vi "Set Status_IO.vi"(8 "error in (no error)":errorcluster, 10 "Status":T1={"Device Data"=variant(cluster{"DeviceName":string, "COM":refnum<visa-resource-name>, "Status String":string, "Input String":string, "DI Value ":i32}[] []), "Ordered ICP1-DO Channels"=[], "Ordered ICP2-DI Channels"=[], "Ordered ICP2-DO Channels"=[], "Ordered ICP1-AI Channels"=[], "Ordered ICP1-AO Channels"=[], "Ordered ICP2-AO Channels"=[]}, 11 "IO in":refnum<class "IO.lvclass">) -> (0 "error out":errorcluster, 3 "IO out":refnum<class "IO.lvclass">)   [LabVIEW 2022 SP3, in "IO.lvclass"]
uses:
  IO.lvclass
  Typedefs/Status Cluster.ctl
  Typedefs/ICP1-D0 Channel Names.ctl
  Typedefs/ICP2-DI Channel Names.ctl
  Typedefs/ICP2-DO Channel Names.ctl
  Typedefs/ICP1-AI Channel Names.ctl
  Typedefs/ICP1-AO Channel Names.ctl
  Typedefs/ICP2-AO Channel Names.ctl
  IO.lvclass/IO.ctl
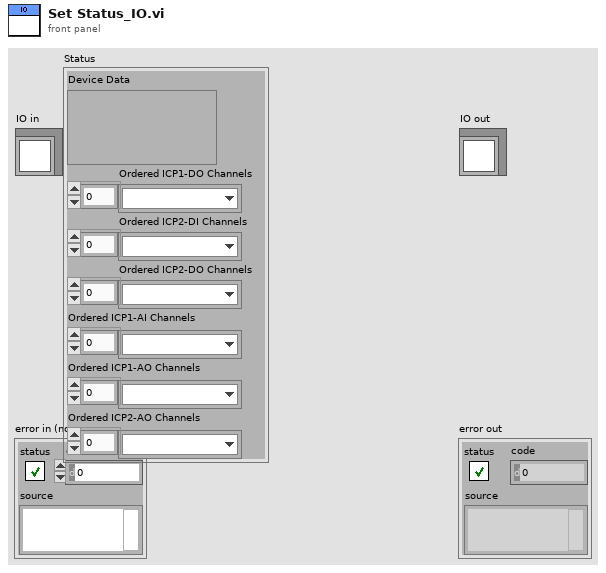
[diagram p1: front panel]
types:
  T1 = typedef "IO.lvclass/Status Cluster.ctl" = cluster{"Device Data":variant, "Ordered ICP1-DO Channels":T2[], "Ordered ICP2-DI Channels":T3[], "Ordered ICP2-DO Channels":T4[], "Ordered ICP1-AI Channels":T5[], "Ordered ICP1-AO Channels":T6[], "Ordered ICP2-AO Channels":T7[]}
  T2 = typedef "IO.lvclass/ICP1-D0 Channel Names.ctl" = enum16{"None", "Meniscus Pressure Reg PWR - R1", "Meniscus Pressure Reg PWR - R2", "Meniscus Pressure Reg PWR - R3", "Meniscus Pressure Reg PWR - R4", "Meniscus Pressure Reg PWR - R5", "Meniscus Pressure Reg PWR - R6", "Clear Stage Alarm", "Servo ON", "Purge Valve Open - R1", "Purge Valve Open - R2", "Purge Valve Open - R3", "Purge Valve Open - R4", "Purge Valve Open - R5", "Purge Valve Open - R6"}
  T3 = typedef "IO.lvclass/ICP2-DI Channel Names.ctl" = enum16{"None", "SW - Ink Valve - R1", "SW - Ink Valve - R2", "SW - Ink Valve - R3", "SW - Ink Valve - R4", "SW - Ink Valve - R5", "SW - Ink Valve - R6", "SW - COVER INPUT SIDE", "SW - COVER OUTPUT SIDE", "SW - Purge - R1", "SW - Purge - R2", "SW - Purge - R3", "SW - Purge - R4", "SW - Purge - R5", "SW - Purge - R6"}
  T4 = typedef "IO.lvclass/ICP2-DO Channel Names.ctl" = enum16{"None", "Meniscus Valve Open - R1", "Meniscus Valve Open - R2", "Meniscus Valve Open - R3", "Meniscus Valve Open - R4", "Meniscus Valve Open - R5", "Meniscus Valve Open - R6", "Ink Flow Valve Open - R1", "Ink Flow Valve Open - R2", "Ink Flow Valve Open - R3", "Ink Flow Valve Open - R4", "Ink Flow Valve Open - R5", "Ink Flow Valve Open - R6", "SW_LED - Ink Valve - R1", "SW_LED - Ink Valve - R2", "SW_LED - Ink Valve - R3", "Recirc Pump On - R1", "Recirc Pump On - R2", "Recirc Pump On - R3", "Recirc Pump On - R4", "Recirc Pump On - R5", "Recirc Pump On - R6", "SW_LED - Ink Valve - R4", "SW_LED - Ink Valve - R5", "SW_LED - Ink Valve - R6"}
  T5 = typedef "IO.lvclass/ICP1-AI Channel Names.ctl" = enum16{"None", "Meniscus Pressure Read - R1", "Meniscus Pressure Read - R2", "Meniscus Pressure Read - R3", "Meniscus Pressure Read - R4", "Meniscus Pressure Read - R5", "Meniscus Pressure Read - R6", "Meniscus Pressure Set - R1", "Meniscus Pressure Set - R2", "Meniscus Pressure Set - R3", "Meniscus Pressure Set - R4", "Meniscus Pressure Set - R5", "Meniscus Pressure Set - R6"}
  T6 = typedef "IO.lvclass/ICP1-AO Channel Names.ctl" = enum16{"None", "Meniscus Pressure Set - R1", "Meniscus Pressure Set - R2", "Meniscus Pressure Set - R3", "Meniscus Pressure Set - R4", "Meniscus Pressure Set - R5", "Meniscus Pressure Set - R6", "Meniscus Vac Pump Speed"}
  T7 = typedef "IO.lvclass/ICP2-AO Channel Names.ctl" = enum16{"None", "Recirc Pump Flow Set - R1", "Recirc Pump Flow Set - R2", "Recirc Pump Flow Set - R3", "Recirc Pump Flow Set - R4", "Recirc Pump Flow Set - R5", "Recirc Pump Flow Set - R6"}
  T8 = typedef "IO.lvclass/Private Data.ctl" = cluster{"UserEvents":T9, "All Dependencies":cluster{"Class References":refnum<class>[], "Class Names":string[]}, "Status":T1}
  T9 = typedef "IO.lvclass/UserEvents.ctl" = cluster{"API Incoming Event":refnum<user-event>, "API Executed Event":refnum<user-event>, "API Return Event":refnum<user-event>, "Status Changed Event":refnum<user-event>}
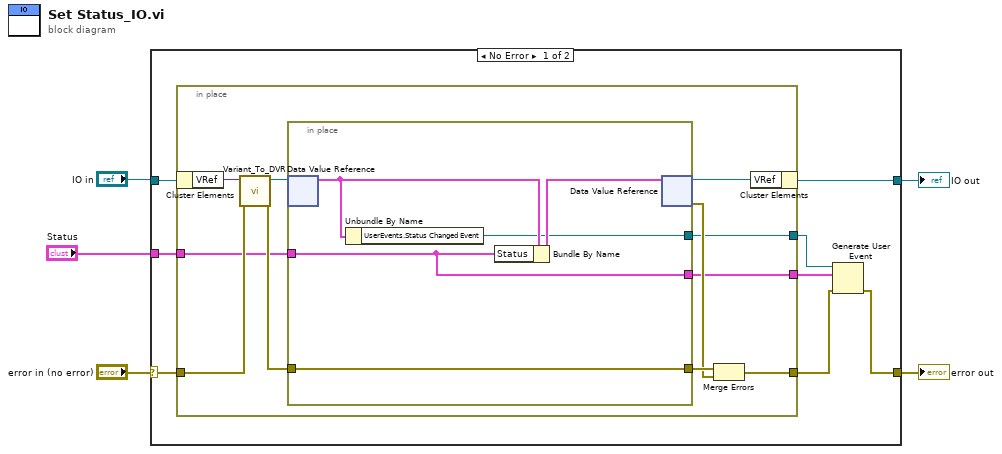
[diagram p0: block diagram]
diagram:
  n1 = case shown="No Error" "error in (no error)" {
    selector: "error in (no error)" -> [w11 w31]
    tunnel: [w6 w31] -> w3
    tunnel: [w13 w30] -> w2
    tunnel: "IO in" -> [w12 w30]
    tunnel: "Status" -> [w10 _]
    frame No Error {
      n2 = in-place {
        in-place-border: w11 -> [w22]
        in-place-border: [w18] -> w7
        in-place-border: w10 -> [w16]
        in-place-border: [w15] -> w9
        in-place-border: [w14] -> w8
        n3 = in-place-cluster #1(w12) -> ("VRef"=w24:variant)
        n4 = call "Variant_To_DVR.vi"("error in (no error)"=w22, "Variant"=w24) -> ("error out"=w21:errorcluster, "DVR"=w23:refnum<data-value>)  [unwired: 8 in]
        n5 = in-place {
          in-place-border: w21 -> [w29]
          in-place-border: [w29] -> w20
          in-place-border: w16 -> [w25]
          in-place-border: [w26] -> w15
          in-place-border: [w25] -> w14
          n6 = in-place-dvr #2(w23) -> (w27:T8)  [unwired: 1 out]
          n7 = Unbundle By Name(w27) -> ("UserEvents.Status Changed Event"=w26:refnum<user-event>)
          n8 = Bundle By Name(cluster=w27, "Status"=w25) -> (w28:T8)
          n9 = in-place-dvr #2(w28) -> (w17:refnum<data-value>, w19:errorcluster)
        }
        n10 = Merge Errors(w20, w19) -> (w18:errorcluster)
        n11 = in-place-cluster #1("VRef"=w17) -> (w13:refnum<class "IO.lvclass">)
      }
      n12 = Generate User Event(user event=w9, event data cluster=w8, error in=w7) -> (error out=w6:errorcluster)  [unwired: 1 in, 1 out]
    }
    frame Error {
    }
  }
  "error out" <- w3
  "IO out" <- w2
